vi "move straight (SubVI).vi"(6 "DST":i32, 8 "error in (no error)":errorcluster, 11 "KNR in":T1) -> (0 "error out":errorcluster, 3 "KNR out":T1)   [LabVIEW 2013]
uses:
  <userlib>/KNR OS 3.0 LabVIEW Toolkit/Type Definition/KNR3 Reference.ctl
  <userlib>/_FPGA Interface Advanced Tools/FPGA Interface Base/FPGA Interface Base.lvclass
  <userlib>/KNR OS 3.0 LabVIEW Toolkit/Type Definition/Resource.ctl
panel:
  in  "STOP":bool
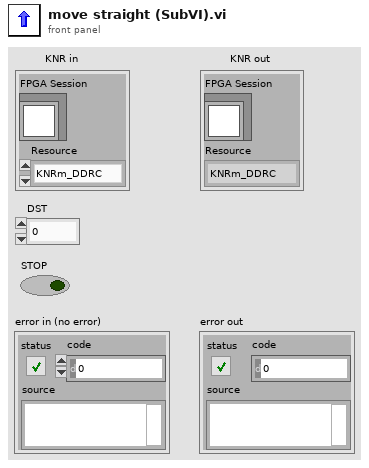
[diagram p1: front panel]
types:
  T1 = typedef "KNR3 Reference.ctl" = cluster{"FPGA Session":refnum<class "FPGA Interface Base.lvclass">, "Resource":T2}
  T2 = typedef "Resource.ctl" = enum16{"KNRm_DDRC", "KNRm_DDDD", "KNRm_DDDR", "KNRm_DDDC", "KNR"}
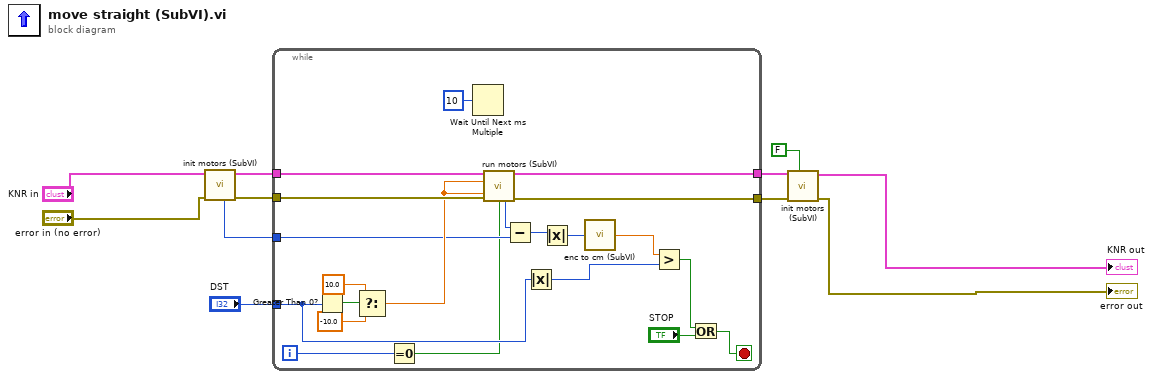
[diagram p0: block diagram]
diagram:
  n1 = call "init motors (SubVI).vi"("error in (no error)"="error in (no error)", "KNR in"="KNR in") -> ("error out"=w2:errorcluster, "KNR out"=w1:T1, "Position_1"=w6:i32)  [unwired: 6 in, 1 out]
  n2 = while {
    tunnel: w1 -> [w32]
    tunnel: w2 -> [w31]
    tunnel: "DST" -> [w24]
    tunnel: [w26] -> w5
    tunnel: [w25] -> w4
    tunnel: w6 -> [w22]
    i -> [w16]
    stop <- w19 stop-if-true
    n3 = Greater Than 0?(x=w24) -> (x > 0?=w30:bool)
    n4 = Select(t=10.0, s=w30, f=-10.0) -> (s? t:f=w27:dbl)
    n5 = Equal To 0?(x=w16) -> (x = 0?=w15:bool)
    n6 = Wait Until Next ms Multiple(millisecond multiple=u32 10) -> ()  [unwired: 1 out]
    n7 = call "run motors (SubVI).vi"("KNR in"=w32, "speed_1"=w27, "speed_2"=w27, "error in (no error)"=w31, "reinitialize? (F)"=w15) -> ("KNR out 2"=w26:T1, "Position_1"=w23:i32, "error out"=w25:errorcluster)  [unwired: 7 in, 1 out]
    n8 = Subtract(x=w23, y=w22) -> (x-y=w21:i32)
    n9 = Absolute Value(x=w24) -> (abs(x)=w20:i32)
    n10 = Absolute Value(x=w21) -> (abs(x)=w13:i32)
    n11 = call "enc to cm (SubVI).vi"("E"=w13) -> ("CM"=w12:dbl)
    n12 = Greater?(x=w12, y=w20) -> (0:w18:bool)
    n13 = Or(x=w18, y="STOP") -> (x .or. y?=w19:bool)
  }
  n14 = call "init motors (SubVI).vi"("Enable Motor(T)"=FALSE, "error in (no error)"=w4, "KNR in"=w5) -> ("error out"=→"error out":errorcluster, "KNR out"=→"KNR out":T1)  [unwired: 5 in, 2 out]
